vi "Digital Pattern Generation.vi"(6 "load data":T5={"max address"=0.0, "memory"="Digital Pattern Gen Memory 0"}, 7 "settings.<user name>":T4, 8 "register bus":T2={"Speed"="Speed", "Crank Angle"="Crank Angle", "Cycle Angle"="Cycle Angle", "Crank Count"="Crank Count", "Cycle Count"="Cycle Count", "1.25 MHz Counter"="1.25 MHz Counter", "Crank Rollover"="Crank Rollover", "Cycle Rollover"="Cycle Rollover", "shared settings"={"start"=0.0, "stuck limit"=0.0}} {"shared settings"."start" format="%#.15g"}, 11 "input.<user name>":T1) -> (2 "digial output":bool)   [LabVIEW 2015, in "Engine Simulation Toolkit.lvlib" / "Digital Pattern Generation.lvlib"]
doc: "Outputs a true or false value depending on engine position and a memory holding positive and negative edges. This is commonly used for hall sensor simulation. <b> This VI should be in an SCTL</b>\n\n<b>settings.<user name></b> - settings for the component. NI VeriStand will set these values. create a control for this input. Replace <user name> with the name you wish this component to display as inside NI VeriStand. Make this name consistent for all controls, indicators, for all VIs of this component.\n<b>input.<user name></b> - input for the component. NI VeriStand will set these values. create a control for this input. Replace <user name> with the name you wish this component to display as inside NI VeriStand. Make this name consistent for all controls, indicators, for all VIs of this component.\n<b>register bus</b> - connect this input to the output of the initialize APU VI. This contains references to APU state variables like position and speed.\n<b>load data</b> - This data comes from Load Digital Pattern Generation.vi\n\n<b>digital output</b> - Wire this to the digital output IO node"
uses:
  Digital Pattern Generation.lvlib
  Load Data.ctl
  Settings.ctl
  APU/Register Bus.ctl
  APU/Shared Settings.ctl
  Input.ctl
  <vilib>/rvi/Emulation/niFpgaSctlEmulationGetInTimedLoop.vi
  <vilib>/Utility/error.llb/Clear Errors.vi
  <vilib>/rvi/DataTransferAndStorage/Container/Common/niFpgaContainerExecOnDevCompGetState.vi
  <vilib>/rvi/Emulation/niFpgaEmulationIsFPGAContextNoSignature.vi
  <vilib>/rvi/DataTransferAndStorage/Container/Common/niFpgaContainerGetUniqueNameForEmu.vi
  <vilib>/rvi/Emulation/niFpgaProcessEmulError.vi
  <vilib>/rvi/errors/nirviReportUnexpectedCaseInternalError (U32).vi
  <vilib>/rvi/Memory/Memory_Emulation/niFpgaMemoryEmulationCacheClearOnFirstRun.vi
  <vilib>/rvi/Memory/Memory_Emulation/nirvimemoryEmulationManagerCache_MakeExclusive.vi
  <vilib>/rvi/Memory/Memory_Emulation/niFpgaMemoryEmulationValidateCache.vi
  <vilib>/rvi/Memory/Memory_Emulation/nirvimemoryEmulationManagerCache_InsertValue.vi
  <vilib>/rvi/Memory/Memory_Emulation/nirvimemoryEmulationManagerCache_ReleaseExclusive.vi
  <vilib>/rvi/Memory/Memory_Emulation/nirvimemoryEmulationManagerCache_GetValue.vi
  <vilib>/rvi/Memory/Memory_Emulation/nirvimemoryEmulationManagerCache_SetValue.vi
  <vilib>/rvi/Emulation/niFpgaSctlEmulationResourceMgr.vi
  <vilib>/rvi/DataTransferAndStorage/Container/XNode/niFpgaContainer.xnode
  <vilib>/rvi/Memory/Memory_Emulation/niFpgaMemoryEmulationRefIn.vi
  APU/APU.lvlib
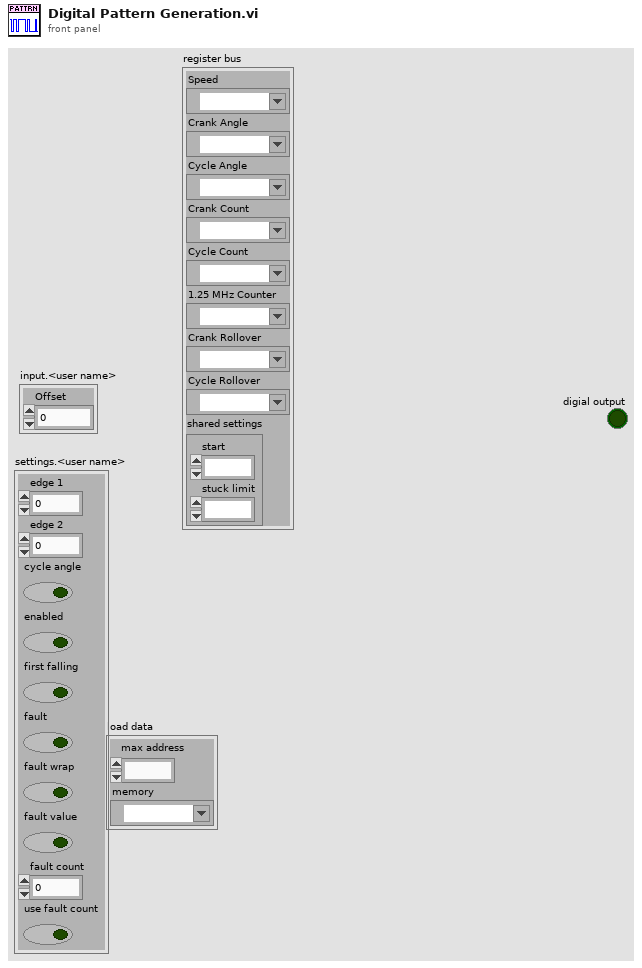
[diagram p1: front panel]
types:
  T1 = typedef "Engine Simulation Toolkit.lvlib/Digital Pattern Generation.lvlib/Input.ctl" = cluster{"Offset":i16}
  T2 = typedef "Engine Simulation Toolkit.lvlib/APU.lvlib/Register Bus.ctl" = cluster{"Speed":refnum<k21>, "Crank Angle":refnum<k21>, "Cycle Angle":refnum<k21>, "Crank Count":refnum<k21>, "Cycle Count":refnum<k21>, "1.25 MHz Counter":refnum<k21>, "Crank Rollover":refnum<k21>, "Cycle Rollover":refnum<k21>, "shared settings":T3}
  T3 = typedef "Engine Simulation Toolkit.lvlib/APU.lvlib/Shared Settings.ctl" = cluster{"start":fxp<+,17,17>, "stuck limit":fxp<+,18,18>}
  T4 = typedef "Engine Simulation Toolkit.lvlib/Digital Pattern Generation.lvlib/Settings.ctl" = cluster{"edge 1":u16, "edge 2":u16, "cycle angle":bool, "enabled":bool, "first falling":bool, "fault":bool, "fault wrap":bool, "fault value":bool, "fault count":fxp<+,4,4>, "use fault count":bool}
  T5 = typedef "Engine Simulation Toolkit.lvlib/Digital Pattern Generation.lvlib/Load Data.ctl" = cluster{"max address":fxp<+,11,11>, "memory":refnum<k21>}
  T6 = typedef "Engine Simulation Toolkit.lvlib/Digital Pattern Generation.lvlib/state data.ctl" = cluster{"output value":bool, "edge 1 value":u16, "edge 2 value":u16, "position to lookup":u16, "edge 1 address":fxp<+,11,11>, "output valid":bool, "wrap":bool, "searching forward":bool, "edge 2 address":fxp<+,11,11>}
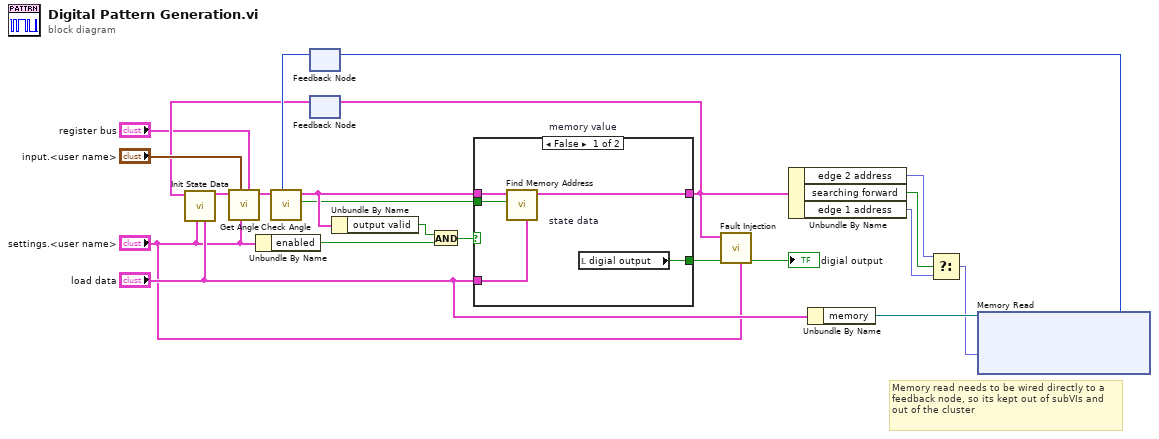
[diagram p0: block diagram]
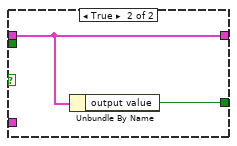
[diagram p2: hidden frame]
diagram:
  # "Memory read needs to be wired directly to a feedback node, so its kept out of subVIs and out of the cluster"
  n1 = Unbundle By Name("settings.<user name>") -> ("enabled"=w18:bool)
  n2 = feedback #1 "memory value"() -> (w14:u16)  [unwired: 1 in]
  n3 = feedback #2 "state data"() -> (w11:T6)  [unwired: 1 in]
  n4 = call "Init State Data.vi"("load data"="load data", "settings.<user name>"="settings.<user name>", "state data in"=w11) -> ("state data out"=w12:T6)  [unwired: 8 in]
  n5 = call "Get Angle.vi"("register bus"="register bus", "settings.<user name>"="settings.<user name>", "input.<user name>"="input.<user name>", "state data in"=w12) -> ("state data out"=w22:T6)  [unwired: 7 in]
  n6 = call "Check Angle.vi"("memory value"=w14, "state data in"=w22) -> (">=edge 1"=w17:bool, "state data out"=w20:T6)  [unwired: 8 in]
  n7 = Unbundle By Name(w20) -> ("output valid"=w21:bool)
  n8 = And(x=w21, y=w18) -> (x .and. y?=w19:bool)
  n9 = case shown="False" w19 {
    tunnel: w20 -> [w26 w28]
    tunnel: [w27 w29] -> w5
    tunnel: [w24 w28] -> w3
    tunnel: "load data" -> [w23 _]
    tunnel: w17 -> [w25 _]
    frame False {
      n10 = call "Find Memory Address.vi"("load data"=w23, ">=edge 1"=w25, "state data in"=w26) -> ("state data out"=w24:T6)  [unwired: 8 in]
      n11 = local read "digial output"() -> (w27:bool)
    }
    frame True {
      n12 = Unbundle By Name(w28) -> ("output value"=w29:bool)
    }
  }
  n13 = feedback-in #2(w3) -> ()
  n14 = call "Fault Injection.vi"("settings.<user name>"="settings.<user name>", "unfaulted DO"=w5, "state data in"=w3) -> ("faulted DO"=→"digial output":bool)  [unwired: 8 in]
  n15 = Unbundle By Name(w3) -> ("edge 2 address"=w9:fxp<+,11,11>, "searching forward"=w10:bool, "edge 1 address"=w6:fxp<+,11,11>)
  n16 = Unbundle By Name("load data") -> ("memory"=w16:refnum<k21>)
  n17 = Select(t=w9, s=w10, f=w6) -> (s? t:f=w8:fxp<+,11,11>)
  n18 = xnode ("Memory Read")("Address"=w8, "Memory In"=w16) -> ("Data"=w15:u16)  [unwired: 1 out]
  n19 = feedback-in #1(w15) -> ()
